vi "emitters 2 PDWs.vi"(8 "error in (no error)":errorcluster, 9 "random startinig phase":bool, 10 "emmiter":T3[](array[typedef]) {"t end" format="%#_3p"; "t start" format="%#_3p"; "DOA" format="%#_3p"}, 11 "device_type in":refnum<class "device_type.lvclass">) -> (0 "error out":errorcluster, 2 "sorted PDWs":T1[](array[typedef]), 3 "device_type out":refnum<class "device_type.lvclass">)   [LabVIEW 2021, in "device_type.lvclass"]
uses:
  device_type.lvclass
  pulse_tx_vis/emitter params.ctl
  pulse_tx_vis/mode_type.ctl
  pulse_tx_vis/PDW_lv2.ctl
  device_type.lvclass/device_type.ctl
  2197b3eb-2394-420c-90e9-03a4284ab46f.vi
  <vilib>/Comparison/Less/Less Functor/Less Functor.lvclass
panel:
  out "may saturate":bool
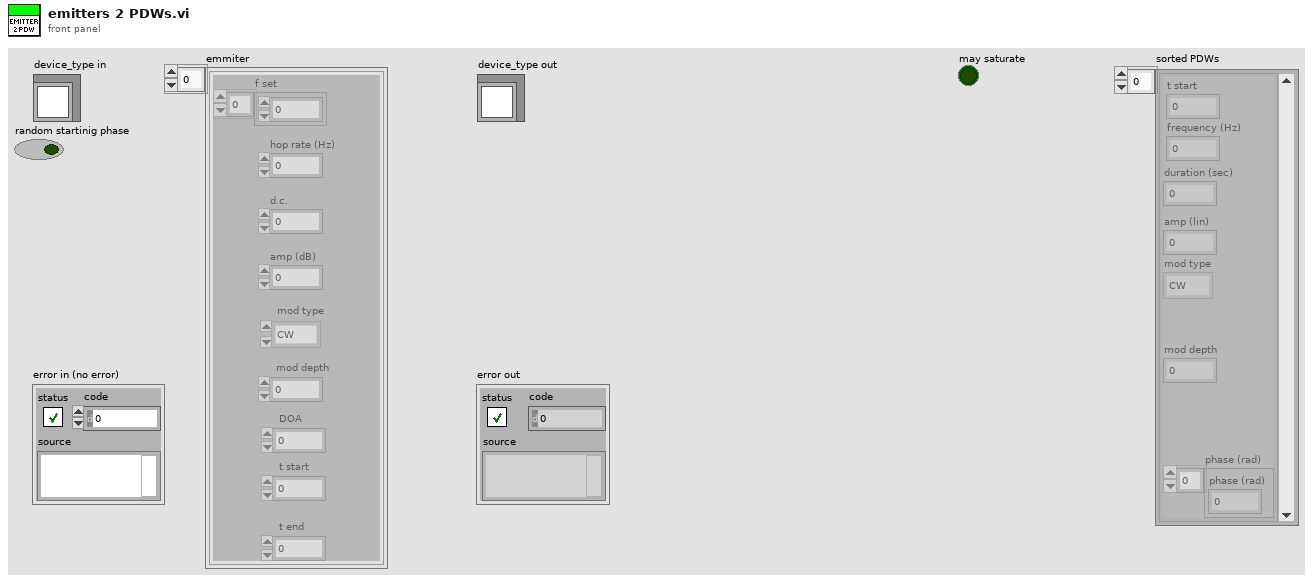
[diagram p1: front panel]
types:
  T1 = typedef "PDW_lv2.ctl" = cluster{"t start":dbl, "frequency (Hz)":dbl, "duration (sec)":dbl, "amp (lin)":dbl, "mod type":T2, "mod depth":dbl, "phase (rad)":dbl[]}
  T2 = typedef "mode_type.ctl" = enum8{"CW", "NC - CW", "NC - cw", "LFM", "BPSK", "QPSK"}
  T3 = typedef "emitter params.ctl" = cluster{"f set":dbl[], "hop rate (Hz)":dbl, "d.c.":dbl, "amp (dB)":dbl, "mod type":T2, "mod depth":dbl, "DOA":dbl, "t start":dbl, "t end":dbl}
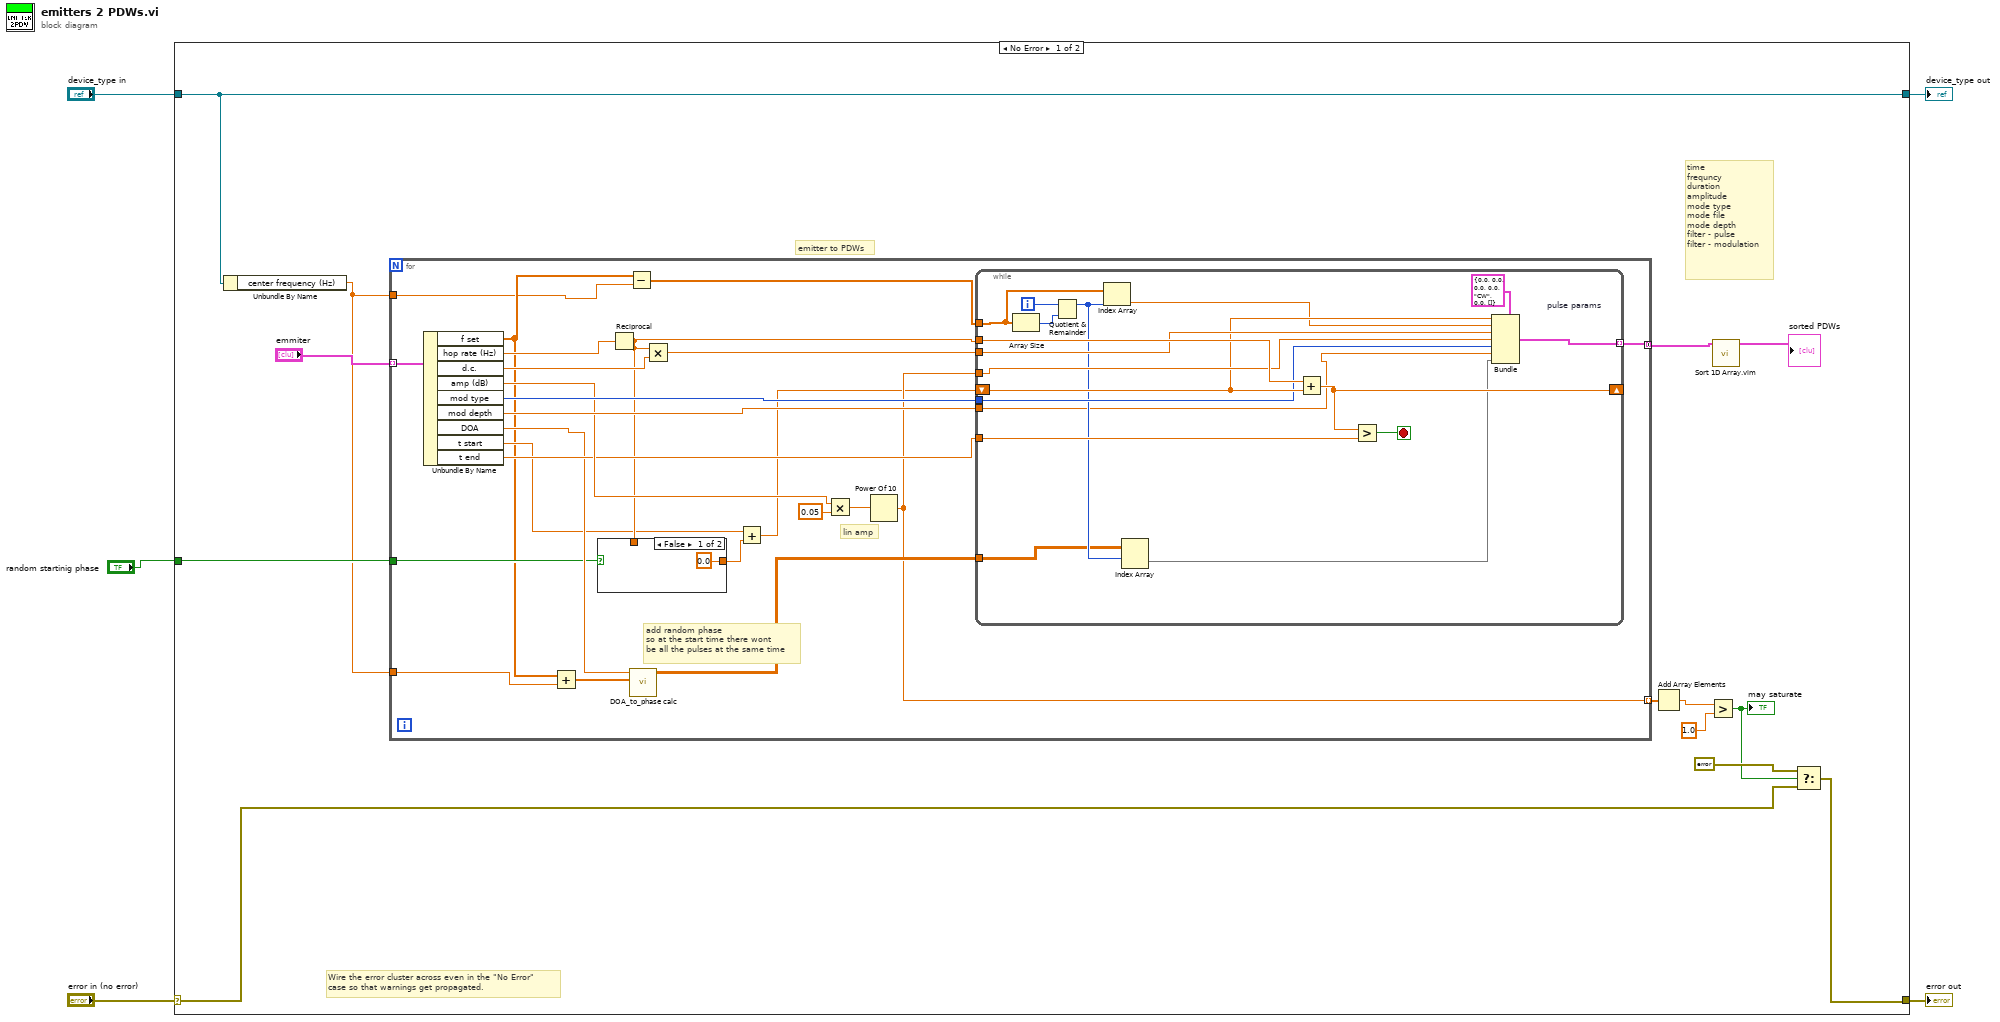
[diagram p0: block diagram]
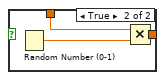
[diagram p2: hidden frame]
diagram:
  n1 = case shown="No Error" "error in (no error)" {
    selector: "error in (no error)" -> [w9 w66]
    tunnel: [w8 w66] -> w4
    tunnel: [w10 w65] -> w2
    tunnel: "device_type in" -> [w10 w65]
    tunnel: "random startinig phase" -> [w7 _]
    frame No Error {
      # "time\nfrequncy\nduration\namplitude\nmode type\nmode file\nmode depth\nfilter - pulse\nfilter - modulation"
      # "emitter to PDWs"
      # "Wire the error cluster across even in the \"No Error\"\ncase so that warnings get propagated."
      n2 = Unbundle By Name(w10) -> ("center frequency (Hz)"=w6:dbl)
      n3 = for {
        tunnel: "emmiter" -> [w42] mode=indexing
        tunnel: [w39] -> w18 mode=concatenating
        tunnel: w6 -> [w29]
        tunnel: [w26] -> w16 mode=indexing
        tunnel: w7 -> [w22]
        tunnel: w6 -> [w20]
        # "add random phase \nso at the start time there wont\nbe all the pulses at the same time"
        # "lin amp"
        n4 = Unbundle By Name(w42) -> ("f set"=w21:dbl[], "hop rate (Hz)"=w36:dbl, "d.c."=w41:dbl, "amp (dB)"=w33:dbl, "mod type"=w38:T2, "mod depth"=w37:dbl, "DOA"=w30:dbl, "t start"=w25:dbl, "t end"=w32:dbl)
        n5 = Add(x=w21, y=w29) -> (x+y=w28:dbl[])
        n6 = Reciprocal(x=w36) -> (1/x=w31:dbl)
        n7 = case shown="False" w22 {
          tunnel: w31 -> [_ w46]
          tunnel: [0.0 w44] -> w24
          frame False {
          }
          frame True {
            n8 = Random Number (0-1)() -> (number: 0 to 1=w45:dbl)
            n9 = Multiply(x=w46, y=w45) -> (x*y=w44:dbl)
          }
        }
        n10 = Subtract(x=w21, y=w20) -> (x-y=w19:dbl[])
        n11 = call "DOA_to_phase calc.vi"("f set (Hz)"=w28, "DOA (deg)"=w30) -> ("phase (rad)"=w27:dbl[][])  [unwired: 9 in]
        n12 = Multiply(x=w31, y=w41) -> (x*y=w40:dbl)
        n13 = Add(x=w25, y=w24) -> (x+y=w23:dbl)
        n14 = Multiply(x=w33, y=0.05) -> (x*y=w34:dbl)
        n15 = Power Of 10(x=w34) -> (10^x=w26:dbl)
        n16 = while {
          tunnel: w19 -> [w62]
          shift-right: [w59] -> _
          shift-left: w23 -> [w54]
          tunnel: w31 -> [w61]
          tunnel: w32 -> [w60]
          tunnel: w40 -> [w57]
          tunnel: w26 -> [w56]
          tunnel: [w55] -> w39 mode=indexing
          tunnel: w38 -> [w52]
          tunnel: w37 -> [w47]
          tunnel: w27 -> [w50]
          i -> [w64]
          stop <- w58 stop-if-true
          n17 = Array Size(array=w62) -> (size(s)=w63:i32)
          n18 = Quotient & Remainder(x=w64, y=w63) -> (x-y*floor(x/y)=w51:i32)  [unwired: 1 out]
          n19 = Index Array(array=w62, index=w51) -> (element=w53:dbl)
          n20 = Index Array(array=w50, index (row)=w51) -> (element=w48:dbl[])  [unwired: 1 in]
          n21 = Add(x=w61, y=w54) -> (x+y=w59:dbl)
          n22 = Greater?(x=w59, y=w60) -> (0:w58:bool)
          n23 = Bundle "pulse params"(cluster=T1 {"t start"=0.0, "frequency (Hz)"=0.0, "duration (sec)"=0.0, "amp (lin)"=0.0, "mod type"=enum."CW", "mod depth"=0.0, "phase (rad)"=[]} ("Cluster"), "t start"=w54, "frequency (Hz)"=w53, "duration (sec)"=w57, "amp (lin)"=w56, "mod type"=w52, "mod depth"=w47, "phase (rad)"=w48) -> (w55:T1)
        }
      }
      n24 = Add Array Elements(numeric array=w16) -> (sum=w15:dbl)
      n25 = Greater?(x=w15, y=1.0) -> (0:w12:bool)
      "may saturate" <- w12
      n26 = call "Sort 1D Array.vim"("unsorted array"=w18) -> ("sorted array"=→"sorted PDWs":T1[])  [unwired: 10 in]
      n27 = Select(t=errorcluster {"status"=FALSE, "code"=5432, "source"="the total amp of all the emmiters are higher then 1, if thay transmit togeder the output will saturate"} ("error out"), s=w12, f=w9) -> (s? t:f=w8:errorcluster)
    }
    frame Error {
    }
  }
  "error out" <- w4
  "device_type out" <- w2
